vi "Queue Driver.vi"(0 "Queue Name":string, 5 "Enqueue Element":T1, 7 "Array of Elements":T1[](array[typedef]), 11 "Error In":errorcluster, 13 "Queue Operation":T2) -> (4 "Dequeue Element":T1, 15 "Error Out":errorcluster)   [LabVIEW 2023]
doc: "The VI performs the queue operations. The operations include create, enqueue, dequeue, flush and closes the queue."
uses:
  Controls/Queue Element.ctl
  Controls/Queue Operation.ctl
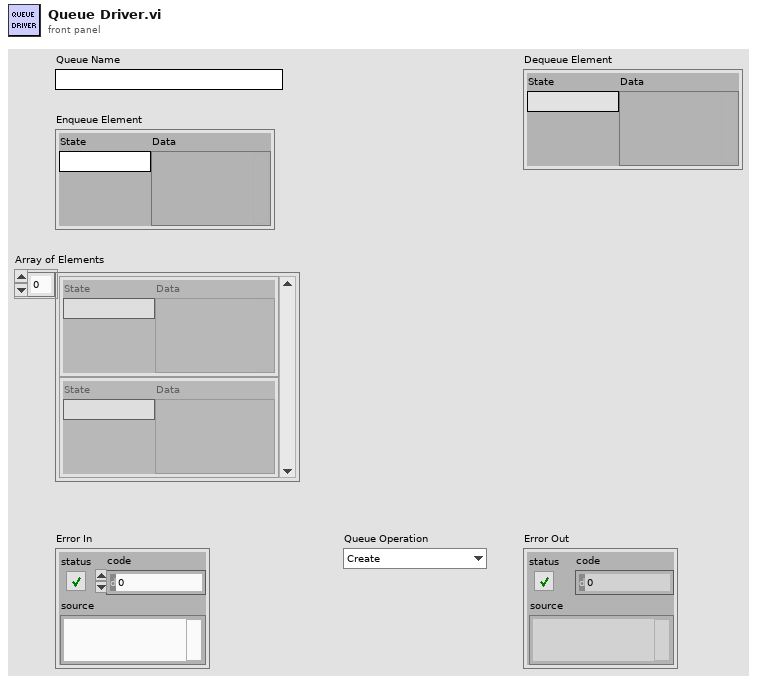
[diagram p1: front panel]
types:
  T1 = typedef "Queue Element.ctl" = cluster{"State":string, "Data":variant}
  T2 = typedef "Queue Operation.ctl" = enum16{"Create", "Enqueue", "Enqueue N", "Dequeue", "Enstack N", "Flush", "Release"}
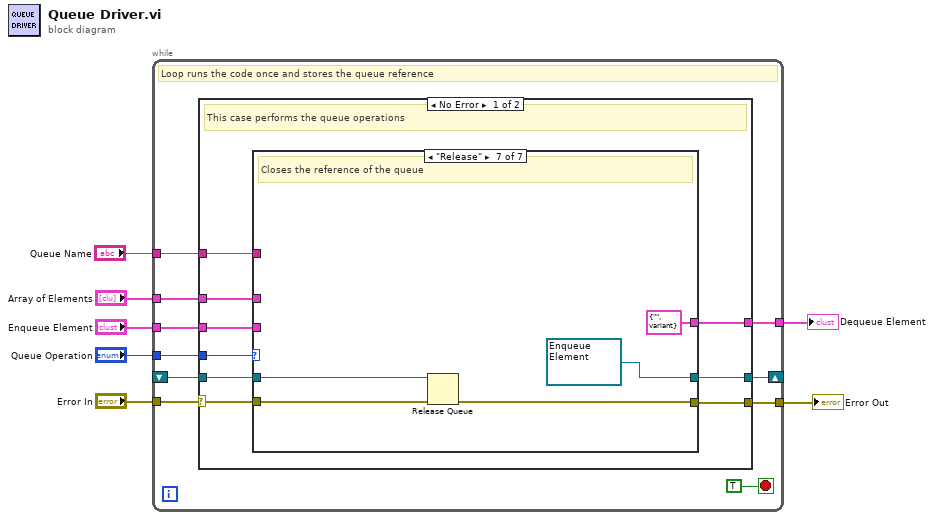
[diagram p0: block diagram]
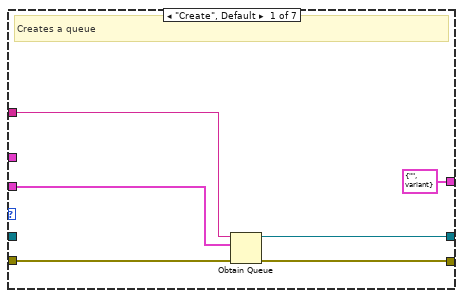
[diagram p2: hidden frame]
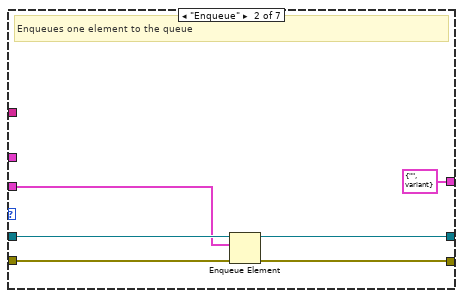
[diagram p3: hidden frame]
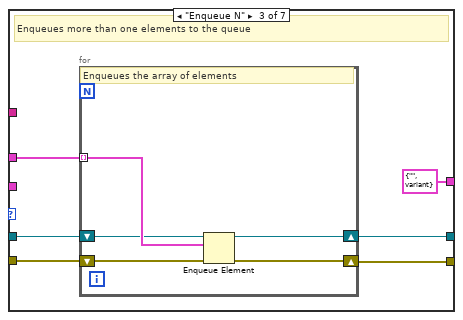
[diagram p4: hidden frame]
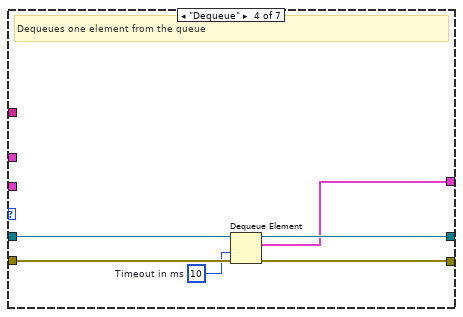
[diagram p5: hidden frame]
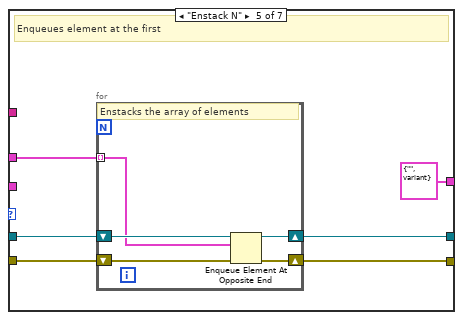
[diagram p6: hidden frame]
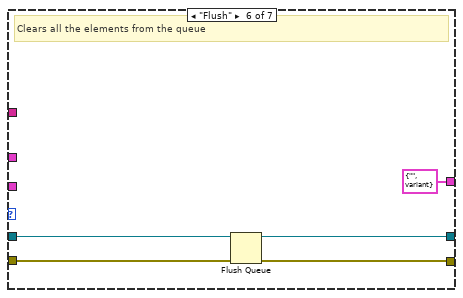
[diagram p7: hidden frame]
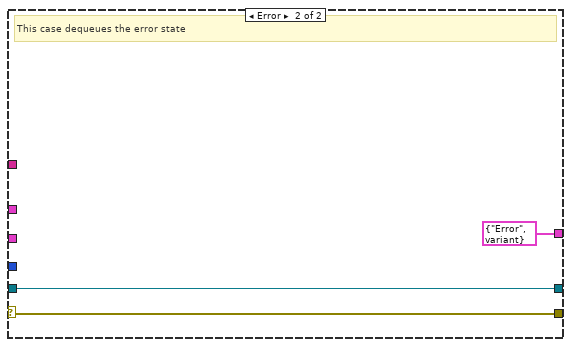
[diagram p8: hidden frame]
diagram:
  n1 = while {
    tunnel: "Error In" -> [w17]
    tunnel: "Queue Operation" -> [w16]
    tunnel: "Queue Name" -> [w15]
    tunnel: "Enqueue Element" -> [w14]
    tunnel: "Array of Elements" -> [w13]
    shift-right: [w12] -> _
    shift-left: _ -> [w11]
    tunnel: [w10] -> w3
    tunnel: [w8] -> w1
    stop <- TRUE stop-if-true
    # "Loop runs the code once and stores the queue reference"
    n2 = case shown="No Error" w17 {
      selector: w17 -> [w26 w78]
      tunnel: w16 -> [w25 _]
      tunnel: w15 -> [w24 _]
      tunnel: w14 -> [w23 _]
      tunnel: w13 -> [w22 _]
      tunnel: [w21 w79] -> w12
      tunnel: w11 -> [w20 w79]
      tunnel: [w19 w78] -> w10
      tunnel: [w18 T1 {"State"="Error", "Data"=variant} ("Enqueue Element")] -> w8
      frame No Error {
        # "This case performs the queue operations"
        n3 = case shown="\"Release\"" w25 {
          tunnel: [w31 w37 w43 w54 w60 w70 w75] -> w19
          tunnel: w26 -> [w32 w38 w44 w55 w61 w71 w76]
          tunnel: w24 -> [w30 _ _ _ _ _ _]
          tunnel: w23 -> [w29 w35 _ _ _ _ _]
          tunnel: w22 -> [_ _ w42 _ w56 _ _]
          tunnel: [w28 w34 w40 w53 w58 w68 refnum<queue> refnum ("queue out")] -> w21
          tunnel: w20 -> [_ w36 w41 w52 w59 w69 w74]
          tunnel: [T1 {"State"="", "Data"=variant} ("Enqueue Element") T1 {"State"="", "Data"=variant} ("Enqueue Element") T1 {"State"="", "Data"=variant} ("Enqueue Element") w50 T1 {"State"="", "Data"=variant} ("Enqueue Element") T1 {"State"="", "Data"=variant} ("Enqueue Element") T1 {"State"="", "Data"=variant} ("Enqueue Element")] -> w18
          frame "Create", Default {
            # "Creates a queue"
            n4 = Obtain Queue(name (unnamed)=w30, element data type=w29, error in (no error)=w32) -> (queue out=w28:refnum<queue>, error out=w31:errorcluster)  [unwired: 2 in, 1 out]
          }
          frame "Enqueue" {
            # "Enqueues one element to the queue"
            n5 = Enqueue Element(queue=w36, element=w35, error in (no error)=w38) -> (queue out=w34:refnum<queue>, error out=w37:errorcluster)  [unwired: 1 in, 1 out]
          }
          frame "Enqueue N" {
            # "Enqueues more than one elements to the queue"
            n6 = for {
              shift-right: [w48] -> w43
              shift-left: w44 -> [w49]
              tunnel: w42 -> [w47] mode=indexing
              shift-right: [w45] -> w40
              shift-left: w41 -> [w46]
              # "Enqueues the array of elements"
              n7 = Enqueue Element(queue=w46, element=w47, error in (no error)=w49) -> (queue out=w45:refnum<queue>, error out=w48:errorcluster)  [unwired: 1 in, 1 out]
            }
          }
          frame "Dequeue" {
            w51 = 10  # Timeout in ms
            # "Dequeues one element from the queue"
            n8 = Dequeue Element(queue=w52, timeout in ms (-1)=w51, error in (no error)=w55) -> (queue out=w53:refnum<queue>, element=w50:T1, error out=w54:errorcluster)  [unwired: 1 out]
          }
          frame "Enstack N" {
            # "Enqueues element at the first"
            n9 = for {
              shift-right: [w65] -> w60
              shift-left: w61 -> [w66]
              shift-right: [w63] -> w58
              shift-left: w59 -> [w64]
              tunnel: w56 -> [w62] mode=indexing
              # "Enstacks the array of elements"
              n10 = Enqueue Element At Opposite End(queue=w64, element=w62, error in (no error)=w66) -> (queue out=w63:refnum<queue>, error out=w65:errorcluster)  [unwired: 1 in, 1 out]
            }
          }
          frame "Flush" {
            # "Clears all the elements from the queue"
            n11 = Flush Queue(queue=w69, error in (no error)=w71) -> (queue out=w68:refnum<queue>, error out=w70:errorcluster)  [unwired: 1 out]
          }
          frame "Release" {
            # "Closes the reference of the queue"
            n12 = Release Queue(queue=w74, error in (no error)=w76) -> (error out=w75:errorcluster)  [unwired: 1 in, 2 out]
          }
        }
      }
      frame Error {
        # "This case dequeues the error state"
      }
    }
  }
  "Error Out" <- w3
  "Dequeue Element" <- w1
